vi "GOOP_MyComputer_Interface_Item_Interface.vi"() -> (3 "InterfaceTable":T1)   [LabVIEW 2020]
uses:
  <resource>/Framework/Providers/API/Item_Interface.ctl
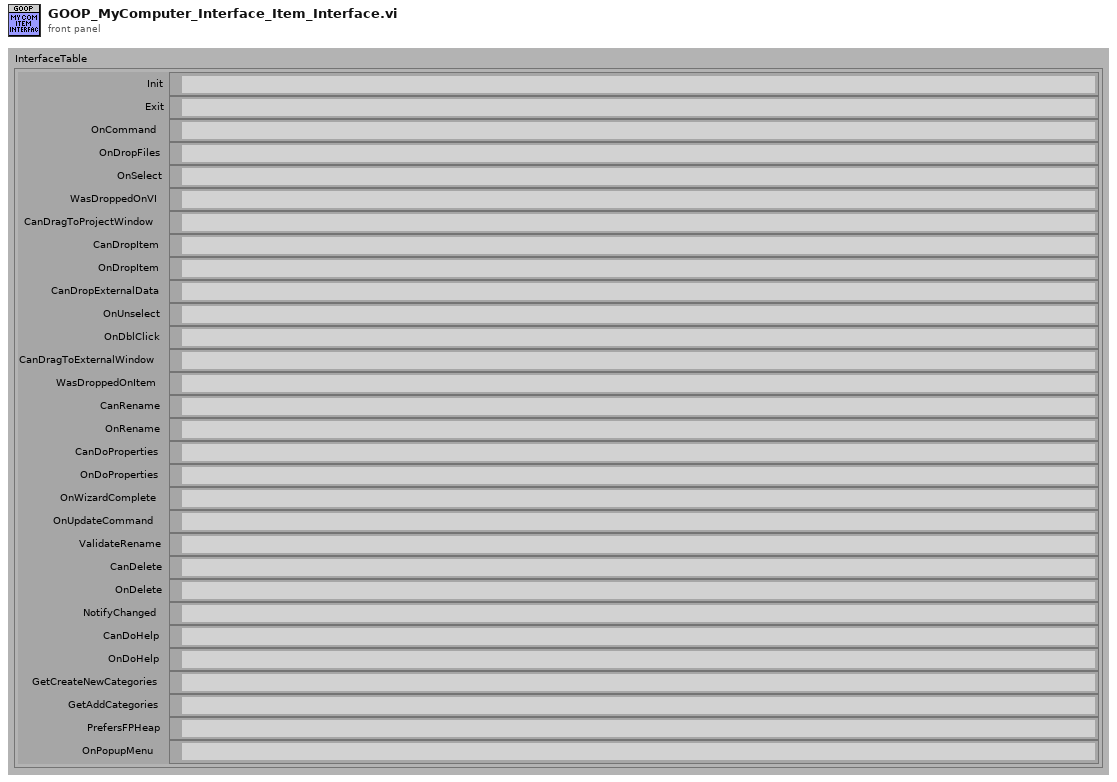
[diagram p1: front panel]
types:
  T1 = typedef "Item_Interface.ctl" = cluster{"Init":path, "Exit":path, "OnCommand":path, "OnDropFiles":path, "OnSelect":path, "WasDroppedOnVI":path, "CanDragToProjectWindow":path, "CanDropItem":path, "OnDropItem":path, "CanDropExternalData":path, "OnUnselect":path, "OnDblClick":path, "CanDragToExternalWindow":path, "WasDroppedOnItem":path, "CanRename":path, "OnRename":path, "CanDoProperties":path, "OnDoProperties":path, "OnWizardComplete":path, "OnUpdateCommand":path, "ValidateRename":path, "CanDelete":path, "OnDelete":path, "NotifyChanged":path, "CanDoHelp":path, "OnDoHelp":path, "GetCreateNewCategories":path, "GetAddCategories":path, "PrefersFPHeap":path, "OnPopupMenu":path}
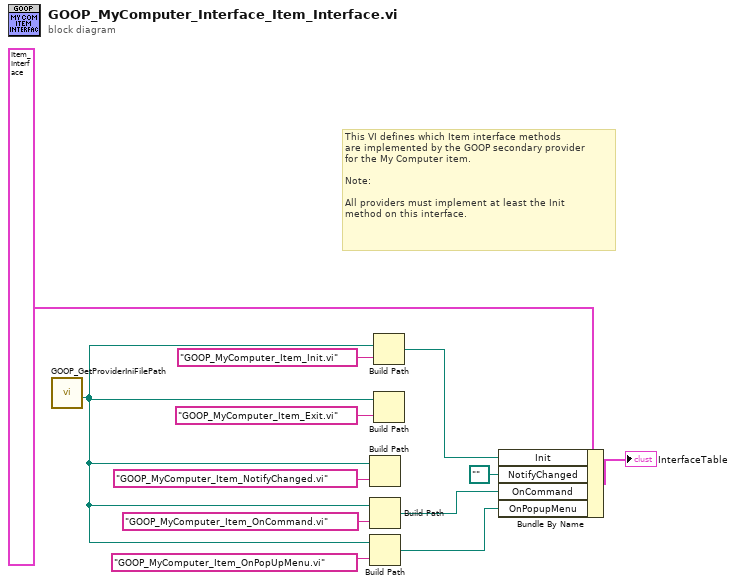
[diagram p0: block diagram]
diagram:
  # "This VI defines which Item interface methods \nare implemented by the GOOP secondary provider \nfor the My Computer item.\n\nNote: \n\nAll providers must implement at least the Init \nmethod on this interface."
  n1 = call <resource>:"GOOP_GetProviderIniFilePath.vi"() -> ("ProviderMainFolder"=w3:path)  [unwired: 10 in, 1 out]
  n2 = Build Path(base path=w3, name or relative path="GOOP_MyComputer_Item_NotifyChanged.vi") -> ()  [unwired: 1 out]
  n3 = Build Path(base path=w3, name or relative path="GOOP_MyComputer_Item_OnCommand.vi") -> (appended path=w6:path)
  n4 = Build Path(base path=w3, name or relative path="GOOP_MyComputer_Item_OnPopUpMenu.vi") -> (appended path=w4:path)
  n5 = Build Path(base path=w3, name or relative path="GOOP_MyComputer_Item_Init.vi") -> (appended path=w10:path)
  n6 = Build Path(base path=w3, name or relative path="GOOP_MyComputer_Item_Exit.vi") -> ()  [unwired: 1 out]
  n7 = Bundle By Name(cluster=T1 {"Init"=path "", "Exit"=path "", "OnCommand"=path "", "OnDropFiles"=path "", "OnSelect"=path "", "WasDroppedOnVI"=path "", "CanDragToProjectWindow"=path "", "CanDropItem"=path "", "OnDropItem"=path "", "CanDropExternalData"=path "", "OnUnselect"=path "", "OnDblClick"=path "", "CanDragToExternalWindow"=path "", "WasDroppedOnItem"=path "", "CanRename"=path "", "OnRename"=path "", "CanDoProperties"=path "", "OnDoProperties"=path "", "OnWizardComplete"=path "", "OnUpdateCommand"=path "", "ValidateRename"=path "", "CanDelete"=path "", "OnDelete"=path "", "NotifyChanged"=path "", "CanDoHelp"=path "", "OnDoHelp"=path "", "GetCreateNewCategories"=path "", "GetAddCategories"=path "", "PrefersFPHeap"=path "", "OnPopupMenu"=path ""} ("InterfaceTable"), "Init"=w10, "NotifyChanged"=path "", "OnCommand"=w6, "OnPopupMenu"=w4) -> (→"InterfaceTable":T1)
